vi "CondimentDecorator_Create.vi"(0 "reference in":refnum<class "CondimentDecorator.lvclass">, 2 "Beverage":refnum<class "Beverage.lvclass">, 3 "CondimentName":string, 5 "error in (no error)":errorcluster) -> (14 "reference out":refnum<class "CondimentDecorator.lvclass">, 19 "error out":errorcluster)   [LabVIEW 2020, in "CondimentDecorator.lvclass"]
uses:
  CondimentDecorator.lvclass
  C:/Projects/OpenGDS_DesignPatterns/Decorator1/Beverage_class/Beverage.lvclass
  Beverage_class/Beverage.lvclass
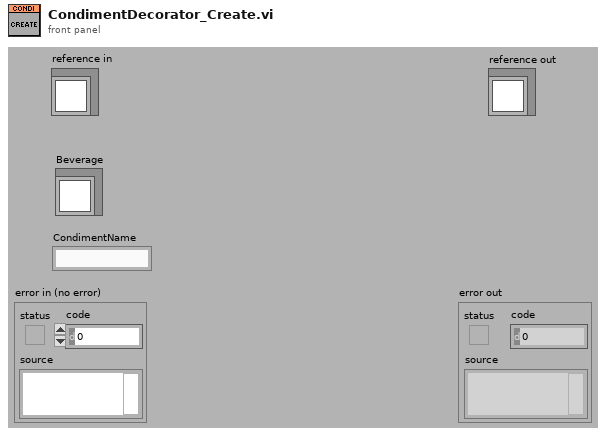
[diagram p1: front panel]
types:
  T1 = typedef "CondimentDecorator.lvclass/ObjectAttributes.ctl" = cluster{"BeverageRef":refnum<class "Beverage.lvclass">, "CondimentName":string}
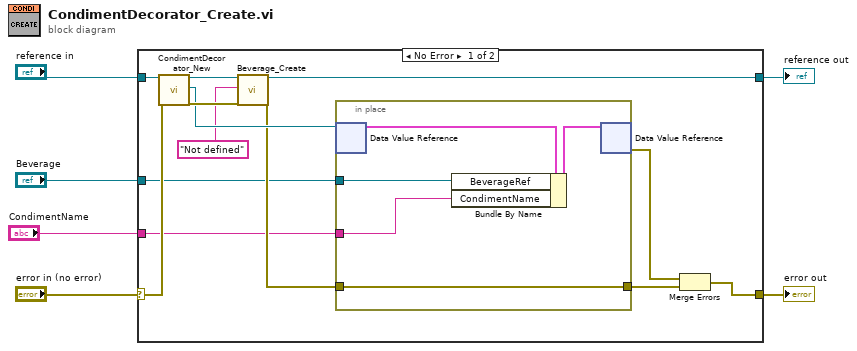
[diagram p0: block diagram]
diagram:
  n1 = case shown="No Error" "error in (no error)" {
    selector: "error in (no error)" -> [w18 w26]
    tunnel: [w16 w26] -> w5
    tunnel: "reference in" -> [w19 w25]
    tunnel: [w13 w25] -> w3
    tunnel: "Beverage" -> [w9 _]
    tunnel: "CondimentName" -> [w7 _]
    frame No Error {
      n2 = call "CondimentDecorator_New.vi"("reference in"=w19, "error in (no error)"=w18) -> ("reference out"=w15:refnum<class "CondimentDecorator.lvclass">, "DVRRefOut"=w12:refnum<data-value>, "error out"=w14:errorcluster)  [unwired: 14 in, 1 out]
      n3 = call "Beverage_Create.vi"("reference in"=w15, "Description"="Not defined", "error in (no error)"=w14) -> ("reference out"=w13:refnum<class "CondimentDecorator.lvclass">, "error out"=w11:errorcluster)  [unwired: 15 in]
      n4 = in-place {
        in-place-border: w11 -> [w22]
        in-place-border: [w22] -> w10
        in-place-border: w9 -> [w21]
        in-place-border: w7 -> [w20]
        n5 = in-place-dvr #1(w12) -> (w23:T1)  [unwired: 1 out]
        n6 = Bundle By Name(cluster=w23, "BeverageRef"=w21, "CondimentName"=w20) -> (w24:T1)
        n7 = in-place-dvr #1(w24) -> (w17:errorcluster)  [unwired: 1 out]
      }
      n8 = Merge Errors(w17, w10) -> (w16:errorcluster)
    }
    frame Error {
    }
  }
  "error out" <- w5
  "reference out" <- w3
